vi "Example_Method.vi"() -> ()   [LabVIEW 2018, in "HttpExamples.lvlib"]
doc: "<b> </b> <b> </b>\nHttpClient_NET\nJustin Young - Viviota\nCopyright (c) 2021\nLicense: BSD"
uses:
  HttpExamples.lvlib
  Types/method_enum.ctl
  HttpHeaders_response/HttpHeaders_Response.lvclass
  C:/Viviota/Projects/R&D/LabVIEW_HTTP_REST_NET/HTTPHeaders_NET/HttpHeaders_NET.lvclass
  HttpHeaders_content/HttpHeaders_Content.lvclass
  <vilib>/httpClient/Base64Encode.vi
  HttpHeaders_Request/HttpHeaders_Request.lvclass
  LabVIEWHTTPClient_NET/HttpClient_NET.lvclass
  HttpContent/HttpContent.lvclass
  HTTPHeaders_NET/HttpHeaders_NET.lvclass
  HttpResponseMessage/HttpResponseMessage.lvclass
  HttpClient_NET.lvlib
  HttpRequestMessage/HttpRequestMessage.lvclass
panel:
  out "Error Out":errorcluster
  in  "timeout_ms (10000)":i32
  in  "ResponseType":enum16{"String", "File", "ByteStream"}(ring)
  out "Content Bytes":string
  out "Timeout":bool
  in  "OutputFilePath":path
  out "ResponseContent Header Values":string[](array[string])
  out "ResponseContent Header Names":string[](array[string])
  in  "error in (no error)":errorcluster
  in  "URL":string="https://reqres.in/api/users?page=2"
  out "Content String":string
  out "Response Header Names":string[](array[string])
  out "Response Header Values":string[](array[string])
  out "StatusCode":i32(ring)=100 items=["Continue"=100, "SwitchingProtocols"=101, "OK"=200, "Created"=201, "Accepted"=202, "NonAuthoritativeInformation"=203, "NoContent"=204, "ResetContent"=205, "PartialContent"=206, "MultipleChoices, Ambiguous"=300, "MovedPermanently, Moved"=301, "Found, Redirect"=302, "SeeOther, RedirectMethod"=303, "NotModified"=304, "UseProxy"=305, "Unused"=306, "TemporaryRedirect, RedirectKeepVerb"=307, "BadRequest"=400, "Unauthorized"=401, "PaymentRequired"=402, "Forbidden"=403, "NotFound"=404, "MethodNotAllowed"=405, "NotAcceptable"=406, "ProxyAuthenticationRequired"=407, "RequestTimeout"=408, "Conflict"=409, "Gone"=410, "LengthRequired"=411, "PreconditionFailed"=412, "RequestEntityTooLarge"=413, "RequestUriTooLong"=414, "UnsupportedMediaType"=415, "RequestedRangeNotSatisfiable"=416, "ExpectationFailed"=417, "UpgradeRequired"=426, "InternalServerError"=500, "NotImplemented"=501, "BadGateway"=502, "ServiceUnavailable"=503, "GatewayTimeout"=504, "HttpVersionNotSupported"=505]
  # "http://httpbin.org/basic-auth/user/password"
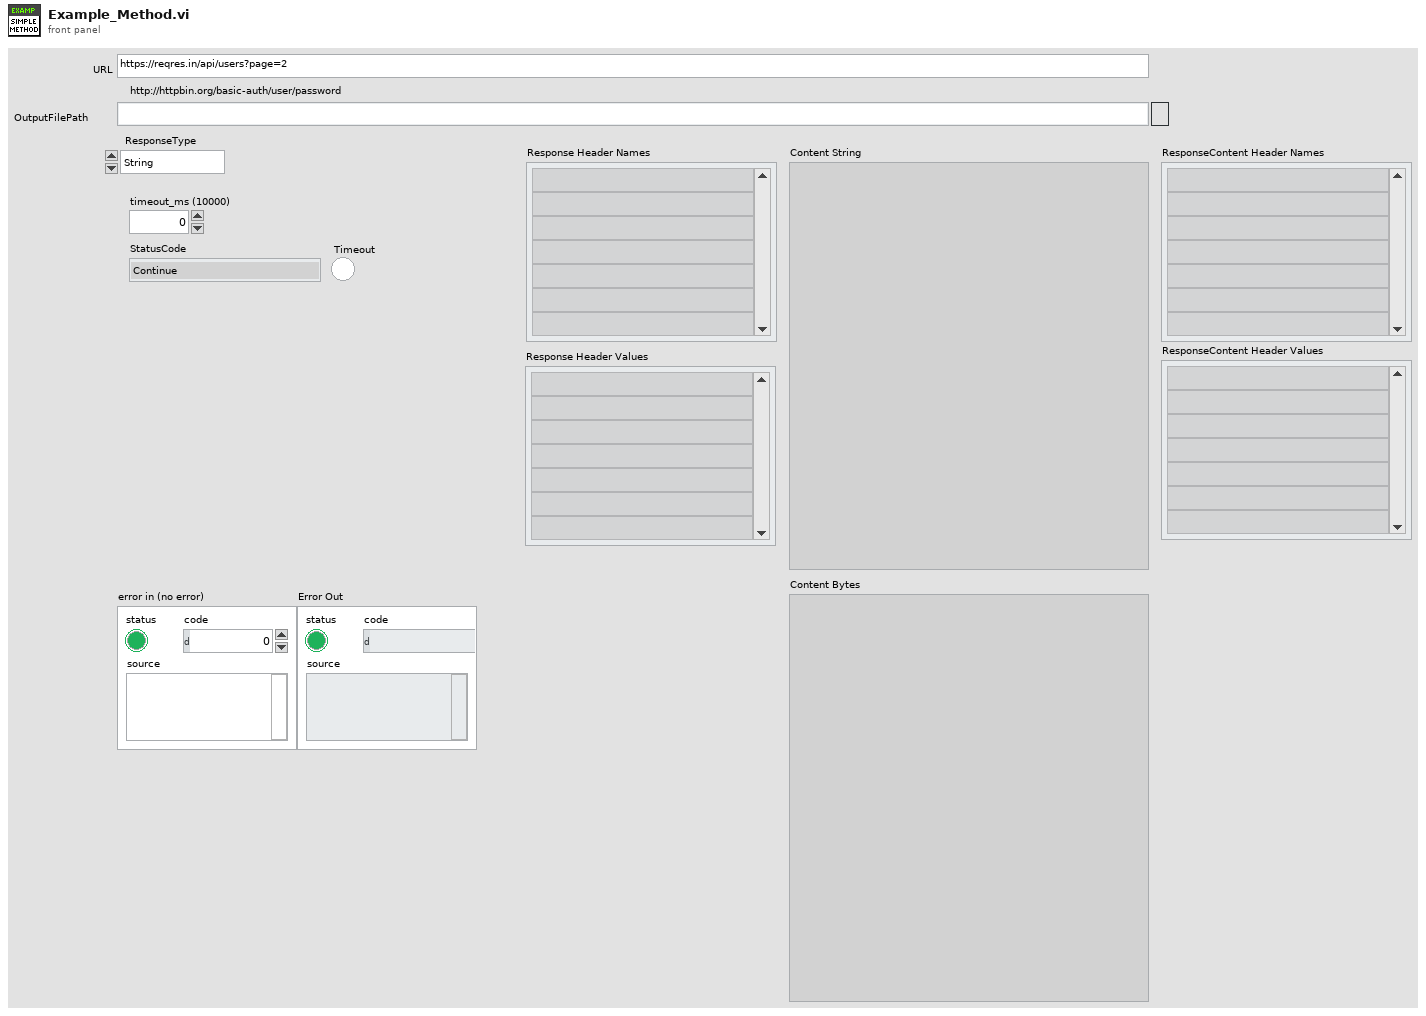
[diagram p1: front panel]
types:
  T1 = typedef "HttpClient_NET.lvlib/method_enum.ctl" = enum16{"GET", "PUT", "POST", "DELETE", "HEAD", "TRACE", "SEND"}
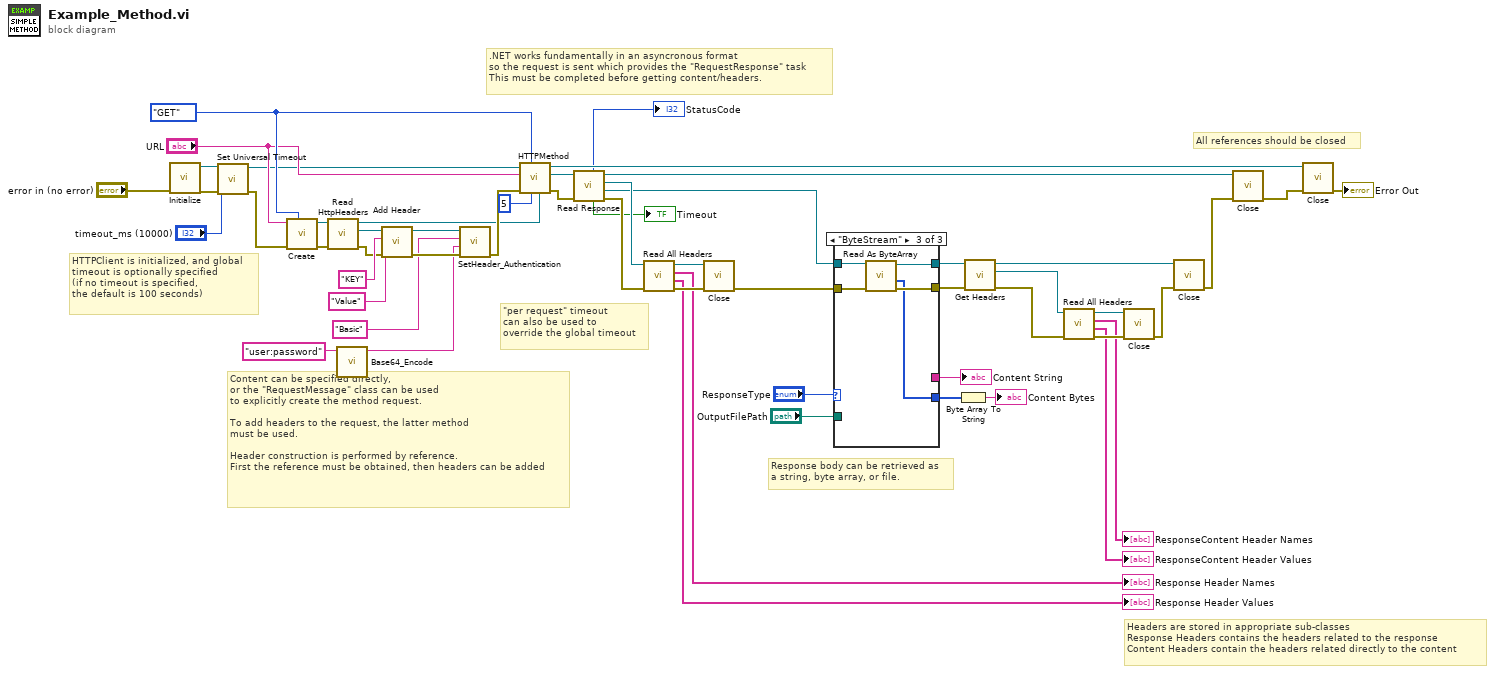
[diagram p0: block diagram]
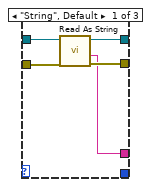
[diagram p2: hidden frame]
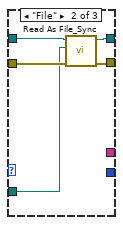
[diagram p3: hidden frame]
diagram:
  w29 = method_enum."GET" ("Method")
  # "Response body can be retrieved as\na string, byte array, or file."
  # "HTTPClient is initialized, and global\ntimeout is optionally specified\n(if no timeout is specified,\nthe default is 100 seconds)"
  # "\"per request\" timeout\ncan also be used to\noverride the global timeout"
  # "All references should be closed"
  # ".NET works fundamentally in an asyncronous format\nso the request is sent which provides the \"RequestResponse\" task\nThis must be completed before getting content/headers."
  # "Headers are stored in appropriate sub-classes\nResponse Headers contains the headers related to the response\nContent Headers contain the headers related directly to the content"
  # "Content can be specified directly, \nor the \"RequestMessage\" class can be used\nto explicitly create the method request.\n\nTo add headers to the request, the latter method\nmust be used.\n\nHeader construction is performed by reference.\nFirst the reference must be obtained, then headers can be added"
  n1 = call "Initialize.vi"("error in (no error)"="error in (no error)") -> ("error out"=w11:errorcluster, "HTTP Client Out"=w14:refnum<class "HttpClient_NET.lvclass">)  [unwired: 9 in]
  n2 = call "Set Universal Timeout.vi"("error in (no error)"=w11, "timeout_ms (10000)"="timeout_ms (10000)", "LabVIEWHTTPClient_NET in"=w14) -> ("error out"=w12:errorcluster, "LabVIEWHTTPClient_NET out"=w13:refnum<class "HttpClient_NET.lvclass">)  [unwired: 7 in]
  n3 = call "Create.vi"("Method [GET]"=w29, "error in (no error)"=w12, "Address"="URL") -> ("error out"=w26:errorcluster, "HttpRequestMessage out"=w27:refnum<class "HttpRequestMessage.lvclass">)  [unwired: 7 in]
  n4 = call "Read HttpHeaders.vi"("error in (no error)"=w26, "HttpRequestMessage in"=w27) -> ("error out"=w23:errorcluster, "HttpHeaders"=w25:refnum<class "HttpHeaders_Request.lvclass">, "HttpRequestMessage out"=w3:refnum<class "HttpRequestMessage.lvclass">)  [unwired: 7 in]
  n5 = call "Base64_Encode.vi"("buffer in"="user:password" ("scheme")) -> ("encoded string"=w16:string)  [unwired: 5 in, 1 out]
  n6 = call-dynamic "Add Header.vi"("error in (no error)"=w23, "Value"="Value", "Name"="KEY", "HTTPHeaders_NET in"=w25) -> ("error out"=w20:errorcluster, "HTTPHeaders_NET out"=w21:refnum<class "HttpHeaders_Request.lvclass">)  [unwired: 6 in]
  n7 = call "SetHeader_Authentication.vi"("error in (no error)"=w20, "parameter"=w16, "scheme"="Basic", "HttpHeaders_Request in"=w21) -> ("error out"=w19:errorcluster)  [unwired: 6 in, 1 out]
  n8 = call "HTTPMethod.vi"("HttpRequestMessage"=w3, "Timeout_ms (10000)"=5, "Method"=w29, "error in (no error)"=w19, "URL"="URL", "LabVIEWHTTPClient_NET in"=w13) -> ("error out"=w34:errorcluster, "HttpResponseMessage out"=w54:refnum<class "HttpResponseMessage.lvclass">, "LabVIEWHTTPClient_NET out"=w48:refnum<class "HttpClient_NET.lvclass">)  [unwired: 3 in]
  n9 = call "Read Response.vi"("error in (no error)"=w34, "HttpResponseMessage in"=w54) -> ("error out"=w33:errorcluster, "HttpContent out"=w7:refnum<class "HttpContent.lvclass">, "HTTPHeaders_NET out"=w51:refnum<class "HttpHeaders_Response.lvclass">, "HttpResponseMessage out"=w49:refnum<class "HttpResponseMessage.lvclass">, "Timeout"=→"Timeout":bool, "StatusCode"=→"StatusCode":i32)  [unwired: 3 in, 1 out]
  n10 = call-dynamic "Read All Headers.vi"("error in (no error)"=w33, "HTTPHeaders_NET in"=w51) -> ("error out"=w52:errorcluster, "Header Values"=→"Response Header Values":string[], "Header Names"=→"Response Header Names":string[], "HTTPHeaders_NET out"=w53:refnum<class "HttpHeaders_Response.lvclass">)  [unwired: 6 in]
  n11 = call "Close.vi"("error in (no error)"=w52, "HTTPHeaders_NET in"=w53) -> ("error out"=w50:errorcluster)  [unwired: 9 in]
  n12 = case shown="\"ByteStream\"" "ResponseType" {
    tunnel: w7 -> [w59 w62 w68]
    tunnel: [w58 w61 w67] -> w44
    tunnel: [w57 w63 w66] -> w43
    tunnel: w50 -> [w56 w64 w69]
    tunnel: "OutputFilePath" -> [_ w60 _]
    tunnel: [w55 _ _] -> w6
    tunnel: [_ _ w65] -> w4
    frame "String", Default {
      n13 = call "Read As String.vi"("error in (no error)"=w56, "HttpContent in"=w59) -> ("error out"=w57:errorcluster, "Content"=w55:string, "HttpContent out"=w58:refnum<class "HttpContent.lvclass">)  [unwired: 7 in]
    }
    frame "File" {
      n14 = call "Read As File_Sync.vi"("error in (no error)"=w64, "FilePath"=w60, "HttpContent in"=w62) -> ("error out"=w63:errorcluster, "HttpContent out"=w61:refnum<class "HttpContent.lvclass">)  [unwired: 4 in, 3 out]
    }
    frame "ByteStream" {
      n15 = call "Read As ByteArray.vi"("error in (no error)"=w69, "HttpContent in"=w68) -> ("error out"=w66:errorcluster, "Content"=w65:u8[], "HttpContent out"=w67:refnum<class "HttpContent.lvclass">)  [unwired: 7 in]
    }
  }
  "Content String" <- w6
  n16 = Byte Array To String(unsigned byte array=w4) -> (string=→"Content Bytes":string)
  n17 = call "Get Headers.vi"("error in (no error)"=w43, "HttpContent in"=w44) -> ("error out"=w40:errorcluster, "HTTPHeaders"=w38:refnum<class "HttpHeaders_Content.lvclass">, "HttpContent out"=w37:refnum<class "HttpContent.lvclass">)  [unwired: 7 in]
  n18 = call-dynamic "Read All Headers.vi"("error in (no error)"=w40, "HTTPHeaders_NET in"=w38) -> ("error out"=w42:errorcluster, "Header Values"=→"ResponseContent Header Values":string[], "Header Names"=→"ResponseContent Header Names":string[], "HTTPHeaders_NET out"=w41:refnum<class "HttpHeaders_Content.lvclass">)  [unwired: 6 in]
  n19 = call "Close.vi"("error in (no error)"=w42, "HTTPHeaders_NET in"=w41) -> ("error out"=w39:errorcluster)  [unwired: 9 in]
  n20 = call "Close.vi"("error in (no error)"=w39, "HttpContent in"=w37) -> ("error out"=w32:errorcluster)  [unwired: 9 in]
  n21 = call "Close.vi"("error in (no error)"=w32, "HttpResponseMessage in"=w49) -> ("error out"=w47:errorcluster)  [unwired: 9 in]
  n22 = call "Close.vi"("Error In"=w47, "LabVIEWHTTPClient_NET in"=w48) -> ("Error Out"=→"Error Out":errorcluster)  [unwired: 9 in]
